vi "Create Log File.vi"(11 "error in (no error)":errorcluster) -> (3 "error out":errorcluster, 4 "Error log refnum out":refnum<file>, 6 "TDMS refnum out":refnum<k34>)   [LabVIEW 2016]
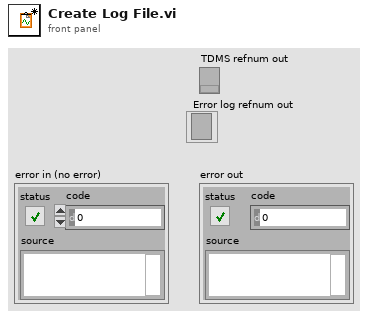
[diagram p1: front panel]
types:
  T1 = enum16{"open", "replace", "create", "open or create", "replace or create", "replace or create with confirmation"}
  T2 = enum16{"open", "open or create", "create or replace", "create", "open (read-only)"}
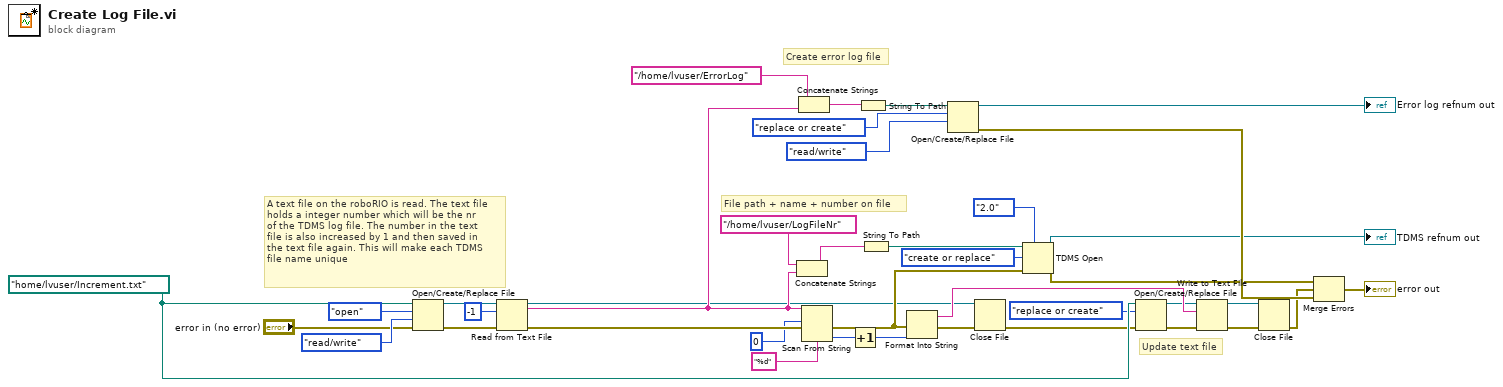
[diagram p0: block diagram]
diagram:
  w11 = path "/home/lvuser/Increment.txt" ("file (use dialog)")
  # "Create error log file"
  # "A text file on the roboRIO is read. The text file\nholds a integer number which will be the nr \nof the TDMS log file. The number in the text \nfile is also increased by 1 and then saved in \nthe text file again. This will make each TDMS \nfile name unique"
  # "Update text file"
  # "File path + name + number on file"
  n1 = Open/Create/Replace File(file path (use dialog)=w11, error in="error in (no error)", operation (0:open)=T1."open", access (0:read/write)=enum16{"read/write", "read-only", "write-only"}."read/write") -> (refnum out=w27:refnum<file>, error out=w23:errorcluster)  [unwired: 2 in, 1 out]
  n2 = Read from Text File(file (use dialog)=w27, count=-1, error in=w23) -> (refnum out=w13:refnum<file>, text=w19:string, error out=w39:errorcluster)  [unwired: 1 in, 1 out]
  n3 = Concatenate Strings("/home/lvuser/LogFileNr" ("string"), w19) -> (w33:string)
  n4 = Concatenate Strings("/home/lvuser/ErrorLog" ("string"), w19) -> (w18:string)
  n5 = Scan From String(format string="%d", input string=w19, initial scan location=u32 0, error in=w39) -> (error out=w22:errorcluster, output 1=w29:i32)  [unwired: 1 in, 2 out]
  n6 = Increment(x=w29) -> (x+1=w28:i32)
  n7 = String To Path(string=w18) -> (path=w17:path)
  n8 = String To Path(string=w33) -> (path=w34:path)
  n9 = Format Into String(error in=w22, w28) -> (resulting string=w30:string, error out=w12:errorcluster)  [unwired: 2 in]
  n10 = Open/Create/Replace File(file path (use dialog)=w17, operation (0:open)=T1."replace or create", access (0:read/write)=enum16{"read/write", "read-only", "write-only"}."read/write") -> (refnum out=→"Error log refnum out":refnum<file>, error out=w14:errorcluster)  [unwired: 3 in, 1 out]
  n11 = Close File(refnum=w13, error in=w12) -> (error out=w6:errorcluster)  [unwired: 1 out]
  n12 = TDMS Open(7:enum16{"1.0", "2.0"}."2.0" ("file format version (2.0)"), 8:w22, 10:T2."create or replace" ("operation (0:open)"), 11:w34) -> (0:w4:errorcluster, 3:→"TDMS refnum out":refnum<k34>)  [unwired: 3 in]
  n13 = Open/Create/Replace File(file path (use dialog)=w11, error in=w6, operation (0:open)=T1."replace or create") -> (refnum out=w10:refnum<file>, error out=w8:errorcluster)  [unwired: 3 in, 1 out]
  n14 = Write to Text File(file (use dialog)=w10, text=w30, error in=w8) -> (refnum out=w9:refnum<file>, error out=w7:errorcluster)  [unwired: 1 in, 1 out]
  n15 = Close File(refnum=w9, error in=w7) -> (error out=w5:errorcluster)  [unwired: 1 out]
  n16 = Merge Errors(w4, w5, w14) -> (→"error out":errorcluster)
